vi "ThLaser_host.vi"() -> ()   [LabVIEW 2013]
uses:
  <instrlib>/niDMM/nidmm.llb/niDMM Configure Measurement Digits.vi
  <instrlib>/niDMM/nidmm.llb/niDMM Resolution in Digits.ctl
  <instrlib>/niDMM/nidmm.llb/niDMM Function.ctl
panel:
  in  "TEC_Source":enum16{"1", "2", "3"}(ring)
  in  "TEC_Channel":enum16{"Ch0", "Ch1", "Ch2"}(ring)=enum."Ch1"
  in  "LD_Source":enum16{"1", "2", "3"}(ring)
  in  "LD_Channel":enum16{"Ch0", "Ch1", "Ch2"}(ring)=enum."Ch1"
  in  "Power Enable":bool
  in  "Установить ток LD":bool
  out "S3_Ch0, V":dbl
  out "S3_Ch2, V":dbl
  out "S3_Ch1, V":dbl
  out "S3_Ch0, mA":dbl
  out "S3_Ch2, mA":dbl
  out "S3_Ch1, mA":dbl
  out "S2_Ch0, V":dbl
  out "S2_Ch2, V":dbl
  out "S2_Ch1, V":dbl
  out "S1_Ch0, V":dbl
  out "S2_Ch0, mA":dbl
  out "S2_Ch2, mA":dbl
  out "S2_Ch1, mA":dbl
  out "S1_Ch0, mA":dbl
  out "4070_address":refnum<k15>="PXI1Slot6_2 (23)" caption="instrument handle out"
  in  "4070":refnum<k15>="PXI1Slot6_2"
  in  "4071(2)":refnum<k15>="PXI1Slot6_2"
  out "4071(2)_address":refnum<k15>="PXI1Slot6_2 (23)" caption="instrument handle out"
  out "4071(1)_address":refnum<k15>="PXI1Slot6_2 (23)" caption="instrument handle out"
  in  "4071(1)":refnum<k15>="PXI1Slot6_2"
  in  "Uпит 3":refnum<k15>="PXI1Slot4"
  out "Vcc(3)_address":refnum<k15>="PXI1Slot4 (3)" caption="instrument handle out"
  in  "Uпит 2":refnum<k15>="PXI1Slot4"
  out "VCC(2)_address":refnum<k15>="PXI1Slot4 (3)" caption="instrument handle out"
  in  "Source":enum16{"1", "2", "Дополнительный"}(ring)
  in  "Channel":enum16{"Channel 0", "Channel 1", "Channel 2"}(ring)
  out "S1_Ch2, V":dbl
  out "S1_Ch1, V":dbl
  in  "Uпит 1":refnum<k15>="PXI1Slot4"
  out "VCC(1)_address":refnum<k15>="PXI1Slot4 (3)" caption="instrument handle out"
  out "S1_Ch2, mA":dbl
  in  "res(input)":dbl=110.0
  in  "Желаемый ток, мА":dbl format="%#_6f"
  in  "Start Voltage":dbl
  in  "stop":bool
  out "S1_Ch1, mA":dbl
  in  "Установить ток Пельтье":bool
  out "Operation":bool
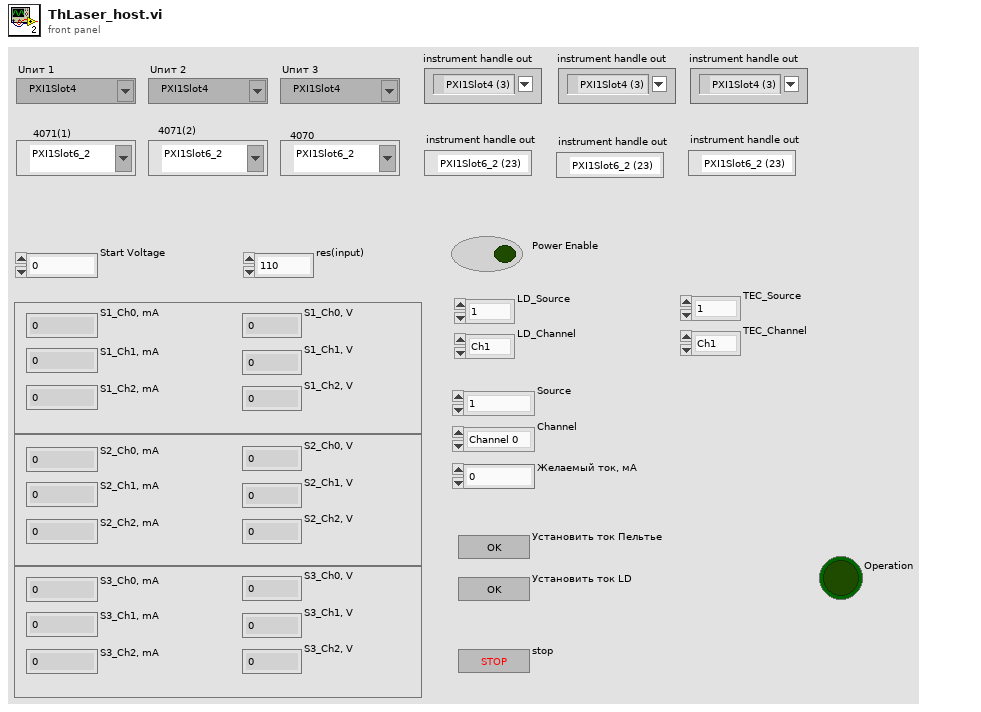
[diagram p1: front panel]
types:
  T1 = cluster{"Case":enum16{"Initialisation", "Idle", "Set Current", "End"}, "Channel":enum16{"Channel 0", "Channel 1", "Channel 2"}, "Source":enum16{"1", "2", "Дополнительный"}}
  T2 = enum16{"Initialisation", "Idle", "Set Current", "End"}
  T3 = typedef "niDMM Function.ctl" = enum16{"DC Volts", "AC Volts", "DC Current", "AC Current", "2-wire Resistance", "4-wire Resistance", "Diode", "Frequency", "Period", "AC Volts DC Coupled", "Capacitance", "Inductance", "Temperature"}
  T4 = typedef "niDMM Resolution in Digits.ctl" = dbl
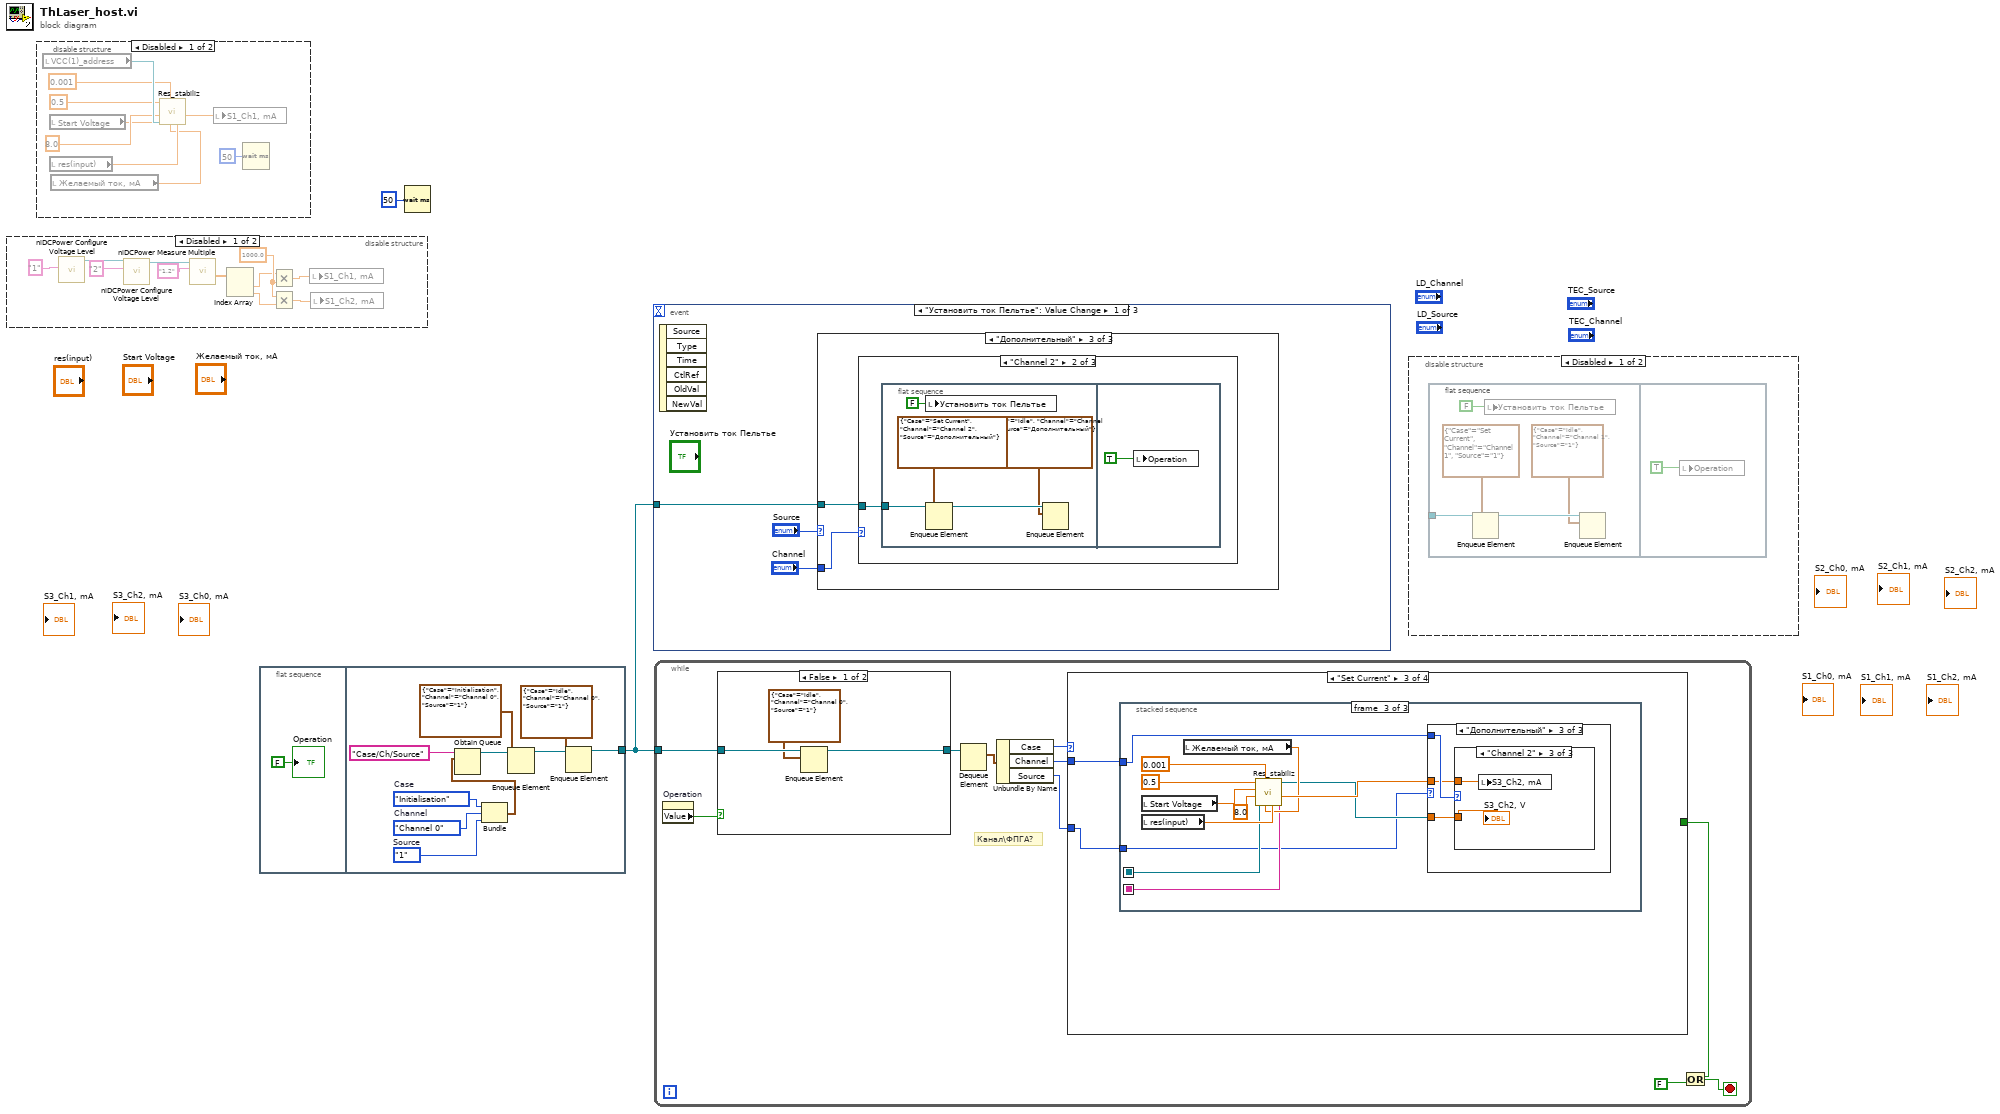
[diagram p0: block diagram]
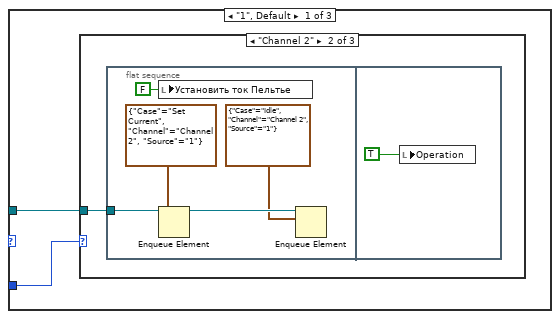
[diagram p5: hidden frame]
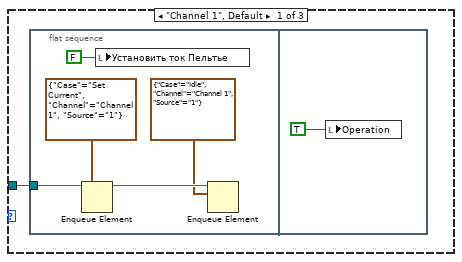
[diagram p6: hidden frame]
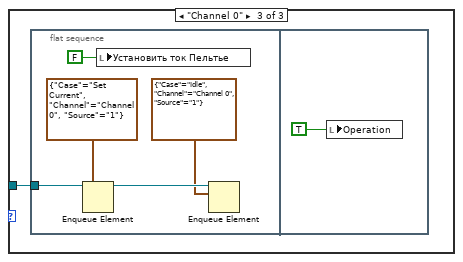
[diagram p7: hidden frame]
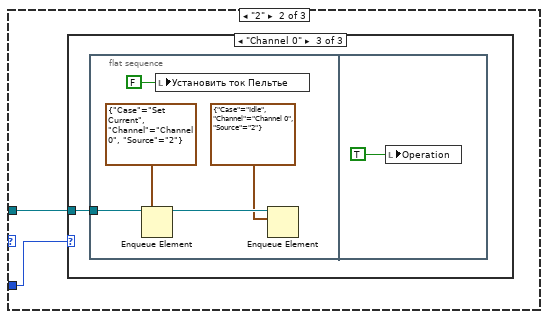
[diagram p8: hidden frame]
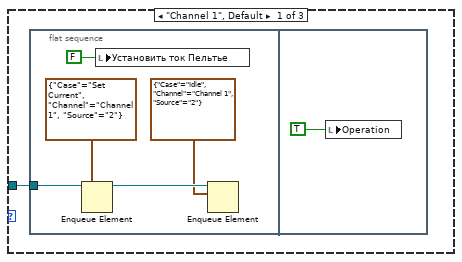
[diagram p9: hidden frame]
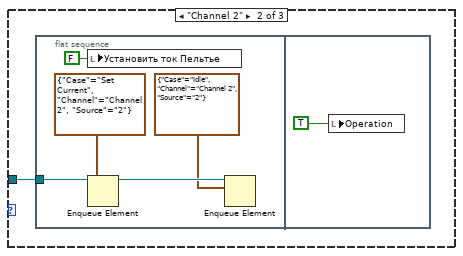
[diagram p10: hidden frame]
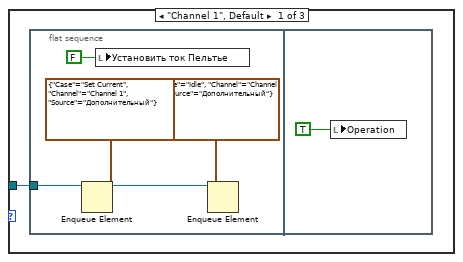
[diagram p11: hidden frame]
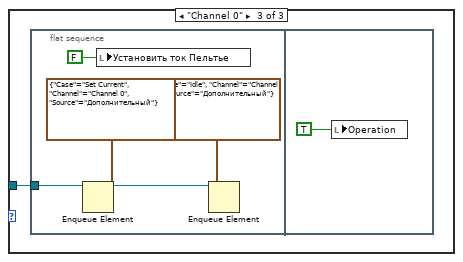
[diagram p12: hidden frame]
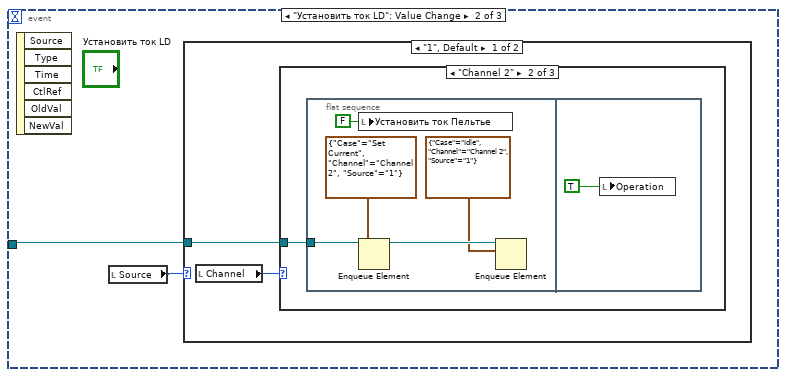
[diagram p13: hidden frame]
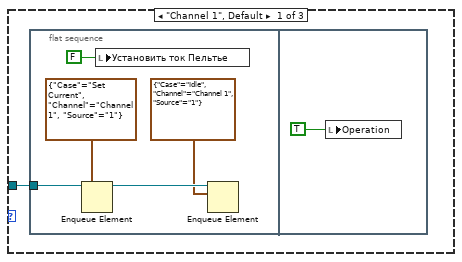
[diagram p14: hidden frame]
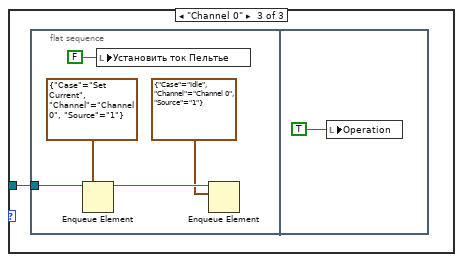
[diagram p15: hidden frame]
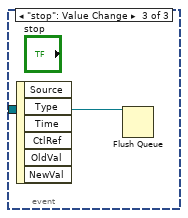
[diagram p17: hidden frame]
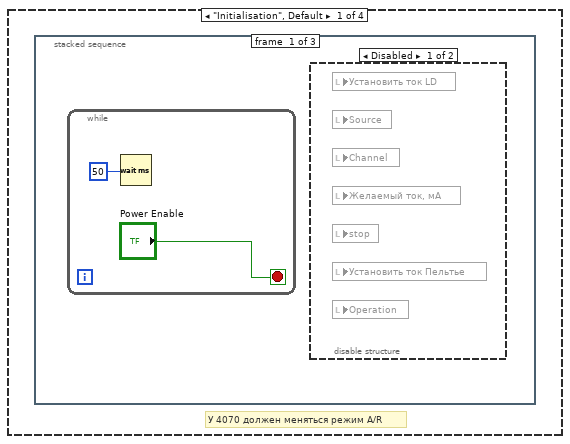
[diagram p18: hidden frame]
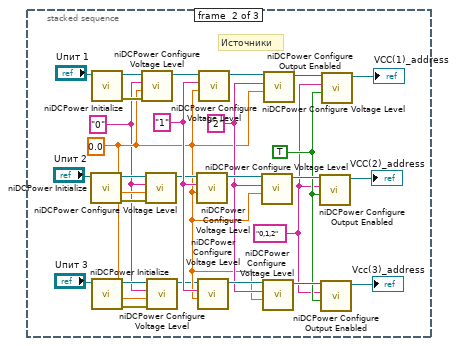
[diagram p20: hidden frame]
diagram:
  n1 = disable-structure shown="Disabled" {
    frame Disabled {
      w13 = 1000.0 ("y")
      n2 = call <instrlib>:"niDCPower Configure Voltage Level.vi"("channel name"="1") -> ("instrument handle out"=w7:refnum<k15>, "voltage level"=w12:dbl)  [unwired: 8 in, 1 out]
      n3 = call <instrlib>:"niDCPower Configure Voltage Level.vi"("channel name"="2", "instrument handle"=w7) -> ("instrument handle out"=w11:refnum<k15>, "voltage level"=w9:dbl)  [unwired: 7 in, 1 out]
      n4 = call <instrlib>:"niDCPower Measure Multiple.vi"("channel name"="1,2", "instrument handle"=w11) -> ("current measurements"=w4:dbl[])  [unwired: 6 in, 3 out]
      n5 = Index Array(array=w4) -> (element #1=w3:dbl, element #2=w10:dbl)  [unwired: 2 in]
      n6 = Multiply(x=w3, y=w13) -> (x*y=w14:dbl)
      n7 = Multiply(x=w13, y=w10) -> (x*y=w15:dbl)
      n8 = local write "S1_Ch1, mA"(w14) -> ()
      n9 = local write "S1_Ch2, mA"(w15) -> ()
    }
    frame Enabled {
    }
  }
  n10 = disable-structure shown="Disabled" {
    frame Disabled {
      n11 = local read "VCC(1)_address"() -> (w24:refnum<k15>)
      n12 = local read "Start Voltage"() -> (w17:dbl)
      n13 = local read "res(input)"() -> (w20:dbl)
      n14 = local read "Желаемый ток, мА"() -> (w19:dbl)
      n15 = call "Res_stabiliz.vi"("res(input)"=w20, "the optimum current(input)"=w19, "accuracy (input)"=0.001, "instrument handle"=w24, "the upper limit for the voltage"=8.0, "Start voltage"=w17, "the lower limit for the voltage"=0.5) -> ("current value, mA"=w22:dbl)  [unwired: 2 in, 2 out]
      n16 = local write "S1_Ch1, mA"(w22) -> ()
      n17 = Wait (ms)(milliseconds to wait=u32 50) -> ()  [unwired: 1 out]
    }
    frame Enabled {
    }
  }
  n18 = flat-sequence {
    tunnel: [w29] -> w2
    frame #0 {
      "Operation" <- FALSE
    }
    frame #1 {
      w28 = enum16{"1", "2", "Дополнительный"}."1"  # Source
      w33 = enum16{"Channel 0", "Channel 1", "Channel 2"}."Channel 0"  # Channel
      w34 = T2."Initialisation"  # Case
      n19 = Bundle("Case"=w34, "Channel"=w33, "Source"=w28) -> (w32:T1)  [unwired: 1 in]
      n20 = Obtain Queue(name (unnamed)="Case/Ch/Source", element data type=w32) -> (queue out=w31:refnum<queue>)  [unwired: 3 in, 2 out]
      n21 = Enqueue Element(queue=w31, element=T1 {"Case"=enum."Initialisation", "Channel"=enum."Channel 0", "Source"=enum."1"}) -> (queue out=w30:refnum<queue>)  [unwired: 2 in, 2 out]
      n22 = Enqueue Element(queue=w30, element=T1 {"Case"=enum."Idle", "Channel"=enum."Channel 0", "Source"=enum."1"}) -> (queue out=w29:refnum<queue>)  [unwired: 2 in, 2 out]
    }
  }
  n23 = Wait (ms)(milliseconds to wait=u32 50) -> ()  [unwired: 1 out]
  n24 = event shown="[0] \"Установить ток Пельтье\": Value Change" {
    selector: _ -> [_ _ _]
    dyn-events: _ -> [_ _ _]
    timeout: _ -> [_ _ _]
    tunnel: w2 -> [w38 w109 w133]
    event "Установить ток Пельтье": Value Change {
      n25 = event-data() -> ()  [unwired: 1 in, 6 out]
      n26 = case shown="\"Дополнительный\"" "Source" {
        tunnel: w38 -> [w40 w63 w86]
        tunnel: "Channel" -> [w39 w62 w85]
        frame "1", Default {
          n27 = case shown="\"Channel 2\"" w39 {
            tunnel: w40 -> [w41 w48 w55]
            frame "Channel 1", Default {
              n28 = flat-sequence {
                tunnel: w41 -> [w46]
                frame #0 {
                  n29 = Enqueue Element(queue=w46, element=T1 {"Case"=enum."Set Current", "Channel"=enum."Channel 1", "Source"=enum."1"}) -> (queue out=w45:refnum<queue>)  [unwired: 2 in, 2 out]
                  n30 = local write "Установить ток Пельтье"(FALSE) -> ()
                  n31 = Enqueue Element(queue=w45, element=T1 {"Case"=enum."Idle", "Channel"=enum."Channel 1", "Source"=enum."1"}) -> ()  [unwired: 2 in, 3 out]
                }
                frame #1 {
                  n32 = local write "Operation"(TRUE) -> ()
                }
              }
            }
            frame "Channel 2" {
              n33 = flat-sequence {
                tunnel: w48 -> [w53]
                frame #0 {
                  n34 = local write "Установить ток Пельтье"(FALSE) -> ()
                  n35 = Enqueue Element(queue=w53, element=T1 {"Case"=enum."Set Current", "Channel"=enum."Channel 2", "Source"=enum."1"}) -> (queue out=w52:refnum<queue>)  [unwired: 2 in, 2 out]
                  n36 = Enqueue Element(queue=w52, element=T1 {"Case"=enum."Idle", "Channel"=enum."Channel 2", "Source"=enum."1"}) -> ()  [unwired: 2 in, 3 out]
                }
                frame #1 {
                  n37 = local write "Operation"(TRUE) -> ()
                }
              }
            }
            frame "Channel 0" {
              n38 = flat-sequence {
                tunnel: w55 -> [w60]
                frame #0 {
                  n39 = Enqueue Element(queue=w60, element=T1 {"Case"=enum."Set Current", "Channel"=enum."Channel 0", "Source"=enum."1"}) -> (queue out=w59:refnum<queue>)  [unwired: 2 in, 2 out]
                  n40 = local write "Установить ток Пельтье"(FALSE) -> ()
                  n41 = Enqueue Element(queue=w59, element=T1 {"Case"=enum."Idle", "Channel"=enum."Channel 0", "Source"=enum."1"}) -> ()  [unwired: 2 in, 3 out]
                }
                frame #1 {
                  n42 = local write "Operation"(TRUE) -> ()
                }
              }
            }
          }
        }
        frame "2" {
          n43 = case shown="\"Channel 0\"" w62 {
            tunnel: w63 -> [w64 w71 w78]
            frame "Channel 1", Default {
              n44 = flat-sequence {
                tunnel: w64 -> [w69]
                frame #0 {
                  n45 = Enqueue Element(queue=w69, element=T1 {"Case"=enum."Set Current", "Channel"=enum."Channel 1", "Source"=enum."2"}) -> (queue out=w68:refnum<queue>)  [unwired: 2 in, 2 out]
                  n46 = local write "Установить ток Пельтье"(FALSE) -> ()
                  n47 = Enqueue Element(queue=w68, element=T1 {"Case"=enum."Idle", "Channel"=enum."Channel 1", "Source"=enum."2"}) -> ()  [unwired: 2 in, 3 out]
                }
                frame #1 {
                  n48 = local write "Operation"(TRUE) -> ()
                }
              }
            }
            frame "Channel 2" {
              n49 = flat-sequence {
                tunnel: w71 -> [w76]
                frame #0 {
                  n50 = local write "Установить ток Пельтье"(FALSE) -> ()
                  n51 = Enqueue Element(queue=w76, element=T1 {"Case"=enum."Set Current", "Channel"=enum."Channel 2", "Source"=enum."2"}) -> (queue out=w75:refnum<queue>)  [unwired: 2 in, 2 out]
                  n52 = Enqueue Element(queue=w75, element=T1 {"Case"=enum."Idle", "Channel"=enum."Channel 2", "Source"=enum."2"}) -> ()  [unwired: 2 in, 3 out]
                }
                frame #1 {
                  n53 = local write "Operation"(TRUE) -> ()
                }
              }
            }
            frame "Channel 0" {
              n54 = flat-sequence {
                tunnel: w78 -> [w83]
                frame #0 {
                  n55 = Enqueue Element(queue=w83, element=T1 {"Case"=enum."Set Current", "Channel"=enum."Channel 0", "Source"=enum."2"}) -> (queue out=w82:refnum<queue>)  [unwired: 2 in, 2 out]
                  n56 = local write "Установить ток Пельтье"(FALSE) -> ()
                  n57 = Enqueue Element(queue=w82, element=T1 {"Case"=enum."Idle", "Channel"=enum."Channel 0", "Source"=enum."2"}) -> ()  [unwired: 2 in, 3 out]
                }
                frame #1 {
                  n58 = local write "Operation"(TRUE) -> ()
                }
              }
            }
          }
        }
        frame "Дополнительный" {
          n59 = case shown="\"Channel 2\"" w85 {
            tunnel: w86 -> [w87 w94 w101]
            frame "Channel 1", Default {
              n60 = flat-sequence {
                tunnel: w87 -> [w92]
                frame #0 {
                  n61 = Enqueue Element(queue=w92, element=T1 {"Case"=enum."Set Current", "Channel"=enum."Channel 1", "Source"=enum."Дополнительный"}) -> (queue out=w91:refnum<queue>)  [unwired: 2 in, 2 out]
                  n62 = local write "Установить ток Пельтье"(FALSE) -> ()
                  n63 = Enqueue Element(queue=w91, element=T1 {"Case"=enum."Idle", "Channel"=enum."Channel 1", "Source"=enum."Дополнительный"}) -> ()  [unwired: 2 in, 3 out]
                }
                frame #1 {
                  n64 = local write "Operation"(TRUE) -> ()
                }
              }
            }
            frame "Channel 2" {
              n65 = flat-sequence {
                tunnel: w94 -> [w99]
                frame #0 {
                  n66 = local write "Установить ток Пельтье"(FALSE) -> ()
                  n67 = Enqueue Element(queue=w99, element=T1 {"Case"=enum."Set Current", "Channel"=enum."Channel 2", "Source"=enum."Дополнительный"}) -> (queue out=w98:refnum<queue>)  [unwired: 2 in, 2 out]
                  n68 = Enqueue Element(queue=w98, element=T1 {"Case"=enum."Idle", "Channel"=enum."Channel 2", "Source"=enum."Дополнительный"}) -> ()  [unwired: 2 in, 3 out]
                }
                frame #1 {
                  n69 = local write "Operation"(TRUE) -> ()
                }
              }
            }
            frame "Channel 0" {
              n70 = flat-sequence {
                tunnel: w101 -> [w106]
                frame #0 {
                  n71 = Enqueue Element(queue=w106, element=T1 {"Case"=enum."Set Current", "Channel"=enum."Channel 0", "Source"=enum."Дополнительный"}) -> (queue out=w105:refnum<queue>)  [unwired: 2 in, 2 out]
                  n72 = local write "Установить ток Пельтье"(FALSE) -> ()
                  n73 = Enqueue Element(queue=w105, element=T1 {"Case"=enum."Idle", "Channel"=enum."Channel 0", "Source"=enum."Дополнительный"}) -> ()  [unwired: 2 in, 3 out]
                }
                frame #1 {
                  n74 = local write "Operation"(TRUE) -> ()
                }
              }
            }
          }
        }
      }
    }
    event "Установить ток LD": Value Change {
      n75 = event-data() -> ()  [unwired: 1 in, 6 out]
      n76 = local read "Source"() -> (w108:enum16{"1", "2", "Дополнительный"})
      n77 = case shown="\"1\", Default" w108 {
        tunnel: w109 -> [w111 _]
        frame "1", Default {
          n78 = local read "Channel"() -> (w110:enum16{"Channel 0", "Channel 1", "Channel 2"})
          n79 = case shown="\"Channel 2\"" w110 {
            tunnel: w111 -> [w112 w119 w126]
            frame "Channel 1", Default {
              n80 = flat-sequence {
                tunnel: w112 -> [w117]
                frame #0 {
                  n81 = Enqueue Element(queue=w117, element=T1 {"Case"=enum."Set Current", "Channel"=enum."Channel 1", "Source"=enum."1"}) -> (queue out=w116:refnum<queue>)  [unwired: 2 in, 2 out]
                  n82 = local write "Установить ток Пельтье"(FALSE) -> ()
                  n83 = Enqueue Element(queue=w116, element=T1 {"Case"=enum."Idle", "Channel"=enum."Channel 1", "Source"=enum."1"}) -> ()  [unwired: 2 in, 3 out]
                }
                frame #1 {
                  n84 = local write "Operation"(TRUE) -> ()
                }
              }
            }
            frame "Channel 2" {
              n85 = flat-sequence {
                tunnel: w119 -> [w124]
                frame #0 {
                  n86 = local write "Установить ток Пельтье"(FALSE) -> ()
                  n87 = Enqueue Element(queue=w124, element=T1 {"Case"=enum."Set Current", "Channel"=enum."Channel 2", "Source"=enum."1"}) -> (queue out=w123:refnum<queue>)  [unwired: 2 in, 2 out]
                  n88 = Enqueue Element(queue=w123, element=T1 {"Case"=enum."Idle", "Channel"=enum."Channel 2", "Source"=enum."1"}) -> ()  [unwired: 2 in, 3 out]
                }
                frame #1 {
                  n89 = local write "Operation"(TRUE) -> ()
                }
              }
            }
            frame "Channel 0" {
              n90 = flat-sequence {
                tunnel: w126 -> [w131]
                frame #0 {
                  n91 = Enqueue Element(queue=w131, element=T1 {"Case"=enum."Set Current", "Channel"=enum."Channel 0", "Source"=enum."1"}) -> (queue out=w130:refnum<queue>)  [unwired: 2 in, 2 out]
                  n92 = local write "Установить ток Пельтье"(FALSE) -> ()
                  n93 = Enqueue Element(queue=w130, element=T1 {"Case"=enum."Idle", "Channel"=enum."Channel 0", "Source"=enum."1"}) -> ()  [unwired: 2 in, 3 out]
                }
                frame #1 {
                  n94 = local write "Operation"(TRUE) -> ()
                }
              }
            }
          }
        }
        frame "2" {
        }
      }
    }
    event "stop": Value Change {
      n95 = event-data() -> ()  [unwired: 1 in, 6 out]
      n96 = Flush Queue(queue=w133) -> ()  [unwired: 1 in, 3 out]
    }
  }
  n97 = while {
    tunnel: w2 -> [w143]
    stop <- w137 stop-if-true
    # "Канал\\ФПГА?"
    n98 = property on="Operation" class="Bool (strict)"() -> ("Value"=w141:bool)  [unwired: 2 in, 2 out]
    n99 = case shown="False" w141 {
      tunnel: w143 -> [w314 w316]
      tunnel: [w313 w315] -> w142
      frame False {
        n100 = Enqueue Element(queue=w314, element=T1 {"Case"=enum."Idle", "Channel"=enum."Channel 0", "Source"=enum."1"}) -> (queue out=w313:refnum<queue>)  [unwired: 2 in, 2 out]
      }
      frame True {
        n101 = Get Queue Status(queue=w316) -> (queue out=w317:refnum<queue>, # elements in queue=w319:i32)  [unwired: 2 in, 6 out]
        n102 = Equal To 0?(x=w319) -> (x = 0?=w318:bool)
        n103 = case shown="True" w318 {
          tunnel: w317 -> [w320 w323]
          tunnel: [w320 w322] -> w315
          frame False {
          }
          frame True {
            n104 = Enqueue Element(queue=w323, element=T1 {"Case"=enum."Initialisation", "Channel"=enum."Channel 0", "Source"=enum."1"}) -> (queue out=w322:refnum<queue>)  [unwired: 2 in, 2 out]
          }
        }
      }
    }
    n105 = Dequeue Element(queue=w142) -> (element=w135:T1)  [unwired: 2 in, 3 out]
    n106 = Unbundle By Name(w135) -> ("Case"=w140:T2, "Channel"=w139:enum16{"Channel 0", "Channel 1", "Channel 2"}, "Source"=w134:enum16{"1", "2", "Дополнительный"})
    n107 = case shown="\"Set Current\"" w140 {
      tunnel: w139 -> [_ _ w252 _]
      tunnel: [_ _ _ w311] -> w136
      tunnel: w134 -> [_ _ w251 _]
      frame "Initialisation", Default {
        # "У 4070 должен меняться режим A/R"
        n108 = stacked-sequence {
          frame #0 {
            n109 = while {
              stop <- "Power Enable" stop-if-true
              n110 = Wait (ms)(milliseconds to wait=50) -> ()  [unwired: 1 out]
            }
            n111 = disable-structure shown="Disabled" {
              frame Disabled {
                n112 = local read "Установить ток LD"() -> ()  [unwired: 1 in]
                n113 = local read "Source"() -> ()  [unwired: 1 in]
                n114 = local read "Channel"() -> ()  [unwired: 1 in]
                n115 = local read "Желаемый ток, мА"() -> ()  [unwired: 1 in]
                n116 = local read "stop"() -> ()  [unwired: 1 in]
                n117 = local read "Установить ток Пельтье"() -> ()  [unwired: 1 in]
                n118 = local read "Operation"() -> ()  [unwired: 1 in]
              }
              frame Enabled {
              }
            }
          }
          frame #1 {
            w146 = "0"
            w160 = TRUE
            w159 = "0,1,2"
            w154 = "2" ("channel name")
            w148 = 0.0 ("voltage level")
            w155 = "1" ("channel name")
            # "Источники"
            n119 = call <instrlib>:"niDCPower Initialize.vi"("resource name"="Uпит 2") -> ("error out"=w152:errorcluster, "instrument handle out"=w153:refnum<k15>)  [unwired: 3 in, 6 out]
            n120 = call <instrlib>:"niDCPower Initialize.vi"("resource name"="Uпит 1") -> ("error out"=w158:errorcluster, "instrument handle out"=w157:refnum<k15>)  [unwired: 3 in, 6 out]
            n121 = call <instrlib>:"niDCPower Initialize.vi"("resource name"="Uпит 3") -> ("error out"=w150:errorcluster, "instrument handle out"=w149:refnum<k15>)  [unwired: 3 in, 6 out]
            n122 = call <instrlib>:"niDCPower Configure Voltage Level.vi"("error in (no error)"=w158, "voltage level"=w148, "channel name"=w146, "instrument handle"=w157) -> ("instrument handle out"=w156:refnum<k15>)  [unwired: 6 in, 1 out]
            n123 = call <instrlib>:"niDCPower Configure Voltage Level.vi"("error in (no error)"=w152, "voltage level"=w148, "channel name"=w146, "instrument handle"=w153) -> ("instrument handle out"=w151:refnum<k15>)  [unwired: 6 in, 1 out]
            n124 = call <instrlib>:"niDCPower Configure Voltage Level.vi"("error in (no error)"=w150, "voltage level"=w148, "channel name"=w146, "instrument handle"=w149) -> ("instrument handle out"=w147:refnum<k15>)  [unwired: 6 in, 1 out]
            n125 = call <instrlib>:"niDCPower Configure Voltage Level.vi"("voltage level"=w148, "channel name"=w155, "instrument handle"=w151) -> ("instrument handle out"=w165:refnum<k15>)  [unwired: 7 in, 1 out]
            n126 = call <instrlib>:"niDCPower Configure Voltage Level.vi"("voltage level"=w148, "channel name"=w155, "instrument handle"=w147) -> ("instrument handle out"=w164:refnum<k15>)  [unwired: 7 in, 1 out]
            n127 = call <instrlib>:"niDCPower Configure Voltage Level.vi"("voltage level"=w148, "channel name"=w155, "instrument handle"=w156) -> ("instrument handle out"=w172:refnum<k15>)  [unwired: 7 in, 1 out]
            n128 = call <instrlib>:"niDCPower Configure Voltage Level.vi"("voltage level"=w148, "channel name"=w154, "instrument handle"=w165) -> ("instrument handle out"=w167:refnum<k15>)  [unwired: 7 in, 1 out]
            n129 = call <instrlib>:"niDCPower Configure Voltage Level.vi"("voltage level"=w148, "channel name"=w154, "instrument handle"=w164) -> ("instrument handle out"=w162:refnum<k15>)  [unwired: 7 in, 1 out]
            n130 = call <instrlib>:"niDCPower Configure Voltage Level.vi"("voltage level"=w148, "channel name"=w154, "instrument handle"=w172) -> ("instrument handle out"=w170:refnum<k15>)  [unwired: 7 in, 1 out]
            n131 = call <instrlib>:"niDCPower Configure Output Enabled.vi"("output enabled"=w160, "channel name"=w159, "instrument handle"=w167) -> ("instrument handle out"=→"VCC(2)_address":refnum<k15>)  [unwired: 7 in, 1 out]
            n132 = call <instrlib>:"niDCPower Configure Output Enabled.vi"("output enabled"=w160, "channel name"=w159, "instrument handle"=w162) -> ("instrument handle out"=→"Vcc(3)_address":refnum<k15>)  [unwired: 7 in, 1 out]
            n133 = call <instrlib>:"niDCPower Configure Output Enabled.vi"("output enabled"=w160, "channel name"=w159, "instrument handle"=w170) -> ("instrument handle out"=→"VCC(1)_address":refnum<k15>)  [unwired: 7 in, 1 out]
          }
          frame #2 {
            w173 = T4 5.5 items=["3 1/2"=3.5, "4 1/2"=4.5, "5 1/2"=5.5, "6 1/2"=6.5, "7 1/2"=7.5] ("Resolution in Digits")
            w175 = TRUE ("Reset")
            w180 = T4 5.5 items=["3 1/2"=3.5, "4 1/2"=4.5, "5 1/2"=5.5, "6 1/2"=6.5, "7 1/2"=7.5] ("Resolution in Digits")
            w182 = TRUE ("Reset")
            w193 = T4 5.5 items=["3 1/2"=3.5, "4 1/2"=4.5, "5 1/2"=5.5, "6 1/2"=6.5, "7 1/2"=7.5] ("Resolution in Digits")
            w191 = TRUE ("Reset")
            # "Мультиметры"
            n134 = call <instrlib>:"niDMM Initialize.vi"("Reset"=w182, "ID Query"=w182, "Instrument Descriptor"="4071(2)") -> ("instrument handle out"=w184:refnum<k15>)  [unwired: 7 in, 1 out]
            n135 = call <instrlib>:"niDMM Initialize.vi"("Reset"=w175, "ID Query"=w175, "Instrument Descriptor"="4070") -> ("instrument handle out"=w177:refnum<k15>)  [unwired: 7 in, 1 out]
            n136 = call <instrlib>:"niDMM Initialize.vi"("Reset"=w191, "ID Query"=w191, "Instrument Descriptor"="4071(1)") -> ("instrument handle out"=w189:refnum<k15>)  [unwired: 7 in, 1 out]
            n137 = call-poly <instrlib>:"niDMM Config Measurement.vi"("Range"=-1.0 ("Configuration:Measurement Options:Max Frequency"), "Resolution in Digits"=w193, "Function"=niDMM_Function."DC Current" ("multimeter mode"), "instrument handle"=w189) -> ("instrument handle out"=w187:refnum<k15>)  [unwired: 6 in, 1 out]
            "4071(1)_address" <- w187
            n138 = call-poly <instrlib>:"niDMM Config Measurement.vi"("Range"=-1.0 ("Configuration:Measurement Options:Max Frequency"), "Resolution in Digits"=w180, "Function"=niDMM_Function."DC Current" ("multimeter mode"), "instrument handle"=w184) -> ("instrument handle out"=w186:refnum<k15>)  [unwired: 6 in, 1 out]
            "4071(2)_address" <- w186
            n139 = call-poly <instrlib>:"niDMM Config Measurement.vi"("Range"=-1.0 ("Configuration:Measurement Options:Max Frequency"), "Resolution in Digits"=w173, "Function"=niDMM_Function."DC Current" ("multimeter mode"), "instrument handle"=w177) -> ("instrument handle out"=w179:refnum<k15>)  [unwired: 6 in, 1 out]
            "4070_address" <- w179
            n140 = call <instrlib>:"niDMM Read.vi"("instrument handle"=w187) -> ()  [unwired: 8 in, 3 out]
            n141 = call <instrlib>:"niDMM Read.vi"("instrument handle"=w186) -> ()  [unwired: 8 in, 3 out]
            n142 = call <instrlib>:"niDMM Read.vi"("instrument handle"=w179) -> ()  [unwired: 8 in, 3 out]
          }
        }
      }
      frame "Idle" {
        w201 = 1000.0 ("y")
        w232 = 1000.0 ("y")
        w235 = 1000.0 ("y")
        n143 = local read "VCC(2)_address"() -> (w198:refnum<k15>)
        n144 = local read "S2_Ch1, V"() -> (w224:dbl)
        n145 = local read "S2_Ch0, V"() -> (w196:dbl)
        n146 = local read "S2_Ch2, V"() -> (w225:dbl)
        n147 = local read "Vcc(3)_address"() -> (w197:refnum<k15>)
        n148 = local read "S1_Ch0, V"() -> (w194:dbl)
        n149 = local read "S3_Ch0, V"() -> (w195:dbl)
        n150 = local read "VCC(1)_address"() -> (w199:refnum<k15>)
        n151 = call <instrlib>:"niDCPower Configure Voltage Level.vi"("voltage level"=w196, "channel name"="0", "instrument handle"=w198) -> ("instrument handle out"=w226:refnum<k15>)  [unwired: 7 in, 1 out]
        n152 = call <instrlib>:"niDCPower Configure Voltage Level.vi"("voltage level"=w194, "channel name"="0", "instrument handle"=w199) -> ("instrument handle out"=w241:refnum<k15>)  [unwired: 7 in, 1 out]
        n153 = call <instrlib>:"niDCPower Configure Voltage Level.vi"("voltage level"=w195, "channel name"="0", "instrument handle"=w197) -> ("instrument handle out"=w207:refnum<k15>)  [unwired: 7 in, 1 out]
        n154 = local read "S1_Ch1, V"() -> (w243:dbl)
        n155 = local read "S3_Ch1, V"() -> (w209:dbl)
        n156 = call <instrlib>:"niDCPower Configure Voltage Level.vi"("voltage level"=w224, "channel name"="1", "instrument handle"=w226) -> ("instrument handle out"=w220:refnum<k15>)  [unwired: 7 in, 1 out]
        n157 = call <instrlib>:"niDCPower Configure Voltage Level.vi"("voltage level"=w243, "channel name"="1", "instrument handle"=w241) -> ("instrument handle out"=w247:refnum<k15>)  [unwired: 7 in, 1 out]
        n158 = call <instrlib>:"niDCPower Configure Voltage Level.vi"("voltage level"=w209, "channel name"="1", "instrument handle"=w207) -> ("instrument handle out"=w213:refnum<k15>)  [unwired: 7 in, 1 out]
        n159 = local read "S1_Ch2, V"() -> (w242:dbl)
        n160 = local read "S3_Ch2, V"() -> (w208:dbl)
        n161 = call <instrlib>:"niDCPower Configure Voltage Level.vi"("voltage level"=w225, "channel name"="2", "instrument handle"=w220) -> ("instrument handle out"=w222:refnum<k15>)  [unwired: 7 in, 1 out]
        n162 = call <instrlib>:"niDCPower Configure Voltage Level.vi"("voltage level"=w242, "channel name"="2", "instrument handle"=w247) -> ("instrument handle out"=w245:refnum<k15>)  [unwired: 7 in, 1 out]
        n163 = call <instrlib>:"niDCPower Configure Voltage Level.vi"("voltage level"=w208, "channel name"="2", "instrument handle"=w213) -> ("instrument handle out"=w211:refnum<k15>)  [unwired: 7 in, 1 out]
        n164 = call <instrlib>:"niDCPower Measure Multiple.vi"("channel name"="0,1,2", "instrument handle"=w222) -> ("current measurements"=w217:dbl[])  [unwired: 6 in, 3 out]
        n165 = call <instrlib>:"niDCPower Measure Multiple.vi"("channel name"="0,1,2", "instrument handle"=w245) -> ("current measurements"=w250:dbl[])  [unwired: 6 in, 3 out]
        n166 = call <instrlib>:"niDCPower Measure Multiple.vi"("channel name"="0,1,2", "instrument handle"=w211) -> ("current measurements"=w216:dbl[])  [unwired: 6 in, 3 out]
        n167 = Index Array(array=w250) -> (element #1=w236:dbl, element #2=w240:dbl, element #3=w239:dbl)  [unwired: 3 in]
        n168 = Index Array(array=w216) -> (element #1=w202:dbl, element #2=w206:dbl, element #3=w205:dbl)  [unwired: 3 in]
        n169 = Index Array(array=w217) -> (element #1=w231:dbl, element #2=w227:dbl, element #3=w228:dbl)  [unwired: 3 in]
        n170 = Multiply(x=w240, y=w235) -> (x*y=w237:dbl)
        n171 = Multiply(x=w235, y=w239) -> (x*y=w244:dbl)
        n172 = Multiply(x=w236, y=w235) -> (x*y=w234:dbl)
        n173 = Multiply(x=w227, y=w232) -> (x*y=w230:dbl)
        n174 = Multiply(x=w232, y=w228) -> (x*y=w223:dbl)
        n175 = Multiply(x=w231, y=w232) -> (x*y=w233:dbl)
        n176 = Multiply(x=w206, y=w201) -> (x*y=w203:dbl)
        n177 = Multiply(x=w201, y=w205) -> (x*y=w210:dbl)
        n178 = Multiply(x=w202, y=w201) -> (x*y=w200:dbl)
        n179 = local write "S1_Ch1, mA"(w237) -> ()
        n180 = local write "S1_Ch0, mA"(w234) -> ()
        n181 = local write "S1_Ch2, mA"(w244) -> ()
        n182 = local write "S2_Ch1, mA"(w230) -> ()
        n183 = local write "S2_Ch0, mA"(w233) -> ()
        n184 = local write "S2_Ch2, mA"(w223) -> ()
        n185 = local write "S1_Ch1, mA"(w203) -> ()
        n186 = local write "S1_Ch0, mA"(w200) -> ()
        n187 = local write "S1_Ch2, mA"(w210) -> ()
      }
      frame "Set Current" {
        n188 = stacked-sequence {
          seq-local: [w253 _ _] -> [_ _ w265]
          seq-local: [_ w258 _] -> [_ _ w264]
          tunnel: w252 -> [_ w259 w266]
          tunnel: w251 -> [w254 _ w263]
          frame #0 {
            n189 = case shown="\"Дополнительный\"" w254 {
              tunnel: [w255 w256 w257] -> w253
              frame "1", Default {
                n190 = local read "VCC(1)_address"() -> (w255:refnum<k15>)
              }
              frame "2" {
                n191 = local read "VCC(2)_address"() -> (w256:refnum<k15>)
              }
              frame "Дополнительный" {
                n192 = local read "Vcc(3)_address"() -> (w257:refnum<k15>)
              }
            }
          }
          frame #1 {
            n193 = case shown="\"Channel 2\"" w259 {
              tunnel: ["1" ("channel name") "2" ("channel name") "0"] -> w258
              frame "Channel 1", Default {
              }
              frame "Channel 2" {
              }
              frame "Channel 0" {
              }
            }
          }
          frame #2 {
            n194 = local read "Start Voltage"() -> (w272:dbl)
            n195 = local read "res(input)"() -> (w271:dbl)
            n196 = local read "Желаемый ток, мА"() -> (w268:dbl)
            n197 = call "Res_stabiliz.vi"("channel name"=w264, "res(input)"=w271, "the optimum current(input)"=w268, "accuracy (input)"=0.001, "instrument handle"=w265, "the upper limit for the voltage"=8.0, "Start voltage"=w272, "the lower limit for the voltage"=0.5) -> ("current value, mA"=w269:dbl, "4070_address"=w267:refnum<k15>)  [unwired: 2 out]
            n198 = case shown="\"Дополнительный\"" w263 {
              tunnel: w269 -> [w277 w284 w294]
              tunnel: w267 -> [w276 w286 w293]
              tunnel: w266 -> [w275 w285 w295]
              frame "1", Default {
                n199 = case shown="\"Channel 1\", Default" w275 {
                  tunnel: w277 -> [w278 w281 w283]
                  tunnel: w276 -> [w279 w280 w282]
                  frame "Channel 0" {
                    n200 = local write "S1_Ch0, mA"(w278) -> ()
                    "S1_Ch0, V" <- w279
                  }
                  frame "Channel 1", Default {
                    n201 = local write "S1_Ch1, mA"(w281) -> ()
                    "S1_Ch1, V" <- w280
                  }
                  frame "Channel 2" {
                    n202 = local write "S1_Ch2, mA"(w283) -> ()
                    "S1_Ch2, V" <- w282
                  }
                }
              }
              frame "2" {
                n203 = case shown="\"Channel 1\", Default" w285 {
                  tunnel: w284 -> [w288 w290 w292]
                  tunnel: w286 -> [w287 w289 w291]
                  frame "Channel 0" {
                    n204 = local write "S1_Ch0, mA"(w288) -> ()
                    "S2_Ch0, V" <- w287
                  }
                  frame "Channel 1", Default {
                    n205 = local write "S2_Ch1, mA"(w290) -> ()
                    "S2_Ch1, V" <- w289
                  }
                  frame "Channel 2" {
                    n206 = local write "S2_Ch2, mA"(w292) -> ()
                    "S2_Ch2, V" <- w291
                  }
                }
              }
              frame "Дополнительный" {
                n207 = case shown="\"Channel 2\"" w295 {
                  tunnel: w294 -> [w297 w299 w301]
                  tunnel: w293 -> [w296 w298 w300]
                  frame "Channel 0", Default {
                    n208 = local write "S3_Ch0, mA"(w297) -> ()
                    "S3_Ch0, V" <- w296
                  }
                  frame "Channel 1" {
                    n209 = local write "S3_Ch1, mA"(w299) -> ()
                    "S3_Ch1, V" <- w298
                  }
                  frame "Channel 2" {
                    n210 = local write "S3_Ch2, mA"(w301) -> ()
                    "S3_Ch2, V" <- w300
                  }
                }
              }
            }
          }
        }
      }
      frame "End" {
        w302 = FALSE
        n211 = local read "VCC(1)_address"() -> (w309:refnum<k15>)
        n212 = local read "VCC(2)_address"() -> (w304:refnum<k15>)
        n213 = local read "Vcc(3)_address"() -> (w303:refnum<k15>)
        n214 = call <instrlib>:"niDCPower Configure Output Enabled.vi"("output enabled"=FALSE, "channel name"="0,1,2", "instrument handle"=w309) -> ()  [unwired: 7 in, 2 out]
        n215 = call <instrlib>:"niDCPower Configure Output Enabled.vi"("output enabled"=FALSE, "channel name"="0,1,2", "instrument handle"=w304) -> ()  [unwired: 7 in, 2 out]
        n216 = call <instrlib>:"niDCPower Configure Output Enabled.vi"("output enabled"=w302, "channel name"="0,1,2", "instrument handle"=w303) -> ()  [unwired: 7 in, 2 out]
        n217 = local write "Power Enable"(w302) -> ()
        n218 = local read "stop"() -> (w311:bool)
      }
    }
    n219 = Or(x=w136, y=FALSE) -> (x .or. y?=w137:bool)
  }
  n220 = disable-structure shown="Disabled" {
    frame Disabled {
      n221 = flat-sequence {
        tunnel: _ -> [w328]
        frame #0 {
          n222 = Enqueue Element(queue=w328, element=T1 {"Case"=enum."Set Current", "Channel"=enum."Channel 1", "Source"=enum."1"}) -> (queue out=w327:refnum<queue>)  [unwired: 2 in, 2 out]
          n223 = local write "Установить ток Пельтье"(FALSE) -> ()
          n224 = Enqueue Element(queue=w327, element=T1 {"Case"=enum."Idle", "Channel"=enum."Channel 1", "Source"=enum."1"}) -> ()  [unwired: 2 in, 3 out]
        }
        frame #1 {
          n225 = local write "Operation"(TRUE) -> ()
        }
      }
    }
    frame Enabled {
    }
  }
